vi "HP-set.vi"(8 "error in (no error)":errorcluster, 10 "write buffer":T1 format="%x", 11 "HP-S-Serial in":refnum<class "HP-S-Serial.lvclass">) -> (0 "error out":errorcluster, 3 "HP-S-Serial out":refnum<class "HP-S-Serial.lvclass">)   [LabVIEW 2020, in "HP-S-Serial.lvclass"]
uses:
  HP-S-Serial.lvclass
  HP-S-data.ctl
  HP-S-Serial.lvclass/HP-S-Serial.ctl
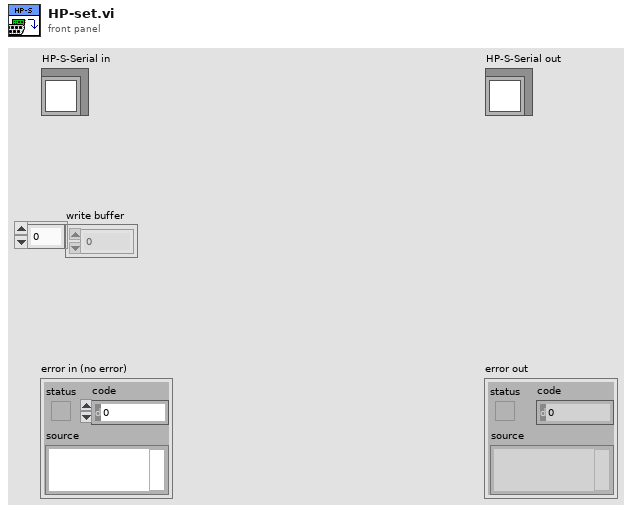
[diagram p1: front panel]
types:
  T1 = typedef "HP-S-Serial.lvclass/HP-S-data.ctl" = u8[]
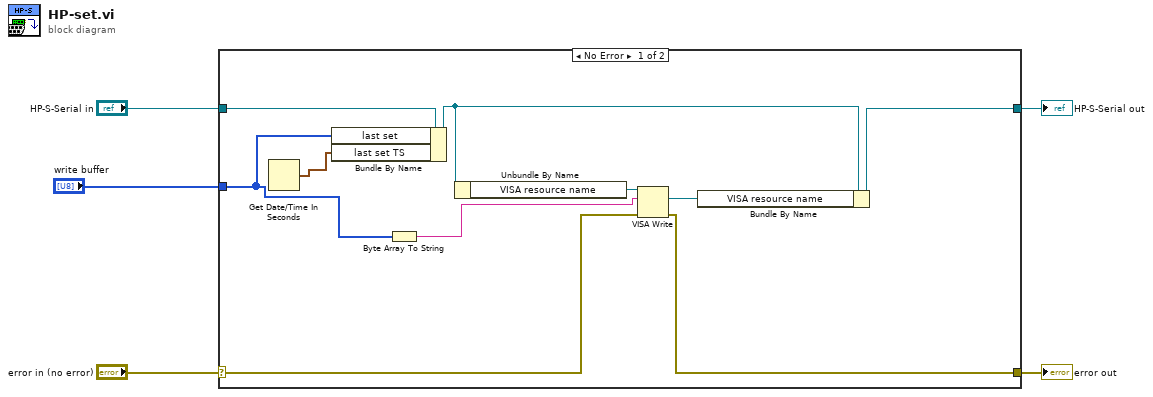
[diagram p0: block diagram]
diagram:
  n1 = case shown="No Error" "error in (no error)" {
    selector: "error in (no error)" -> [w11 w17]
    tunnel: [w10 w17] -> w4
    tunnel: [w15 w16] -> w2
    tunnel: "HP-S-Serial in" -> [w13 w16]
    tunnel: "write buffer" -> [w7 _]
    frame No Error {
      n2 = Get Date/Time In Seconds() -> (seconds since 1Jan1904=w8:timestamp)
      n3 = Bundle By Name(cluster=w13, "last set"=w7, "last set TS"=w8) -> (w9:refnum<class "HP-S-Serial.lvclass">)
      n4 = Byte Array To String(unsigned byte array=w7) -> (string=w6:string)
      n5 = Unbundle By Name(w9) -> ("VISA resource name"=w12:refnum<visa-resource-name>)
      n6 = VISA Write(VISA resource name=w12, write buffer=w6, error in (no error)=w11) -> (VISA resource name out=w14:refnum<visa-resource-name>, error out=w10:errorcluster)  [unwired: 1 out]
      n7 = Bundle By Name(cluster=w9, "VISA resource name"=w14) -> (w15:refnum<class "HP-S-Serial.lvclass">)
    }
    frame Error {
    }
  }
  "error out" <- w4
  "HP-S-Serial out" <- w2
